vi "case.vi"() -> ()   [LabVIEW 2018]
panel:
  in  "Enum":enum16{"random", "1", "0"}(ring)
  out "number: 0 to 1":dbl(graph)
  in  "stop":bool
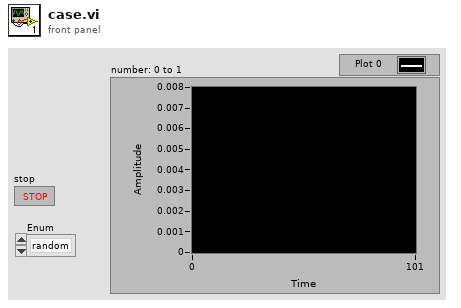
[diagram p1: front panel]
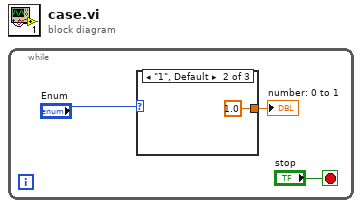
[diagram p0: block diagram]
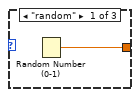
[diagram p2: hidden frame]
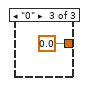
[diagram p3: hidden frame]
diagram:
  n1 = while {
    stop <- "stop" stop-if-true
    n2 = case shown="\"1\", Default" "Enum" {
      tunnel: [w4 1.0 ("number: 0 to 1") 0.0 ("number: 0 to 1")] -> w2
      frame "random" {
        n3 = Random Number (0-1)() -> (number: 0 to 1=w4:dbl)
      }
      frame "1", Default {
      }
      frame "0" {
      }
    }
    "number: 0 to 1" <- w2
  }
